vi "Treat Frame Name for Dialog.vi"(9 "Selected Structure":T1, 10 "index of element":i32, 11 "Frame Name (tag)":string) -> (3 "Frame Name for Dialog":string)   [LabVIEW 2020]
uses:
  StructureTypes.ctl
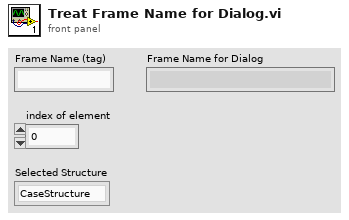
[diagram p1: front panel]
types:
  T1 = typedef "StructureTypes.ctl" = enum16{"CaseStructure", "EventStructure"}
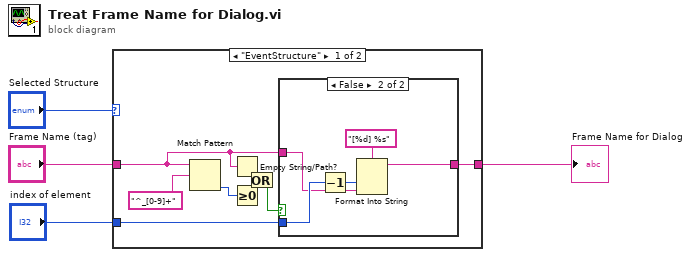
[diagram p0: block diagram]
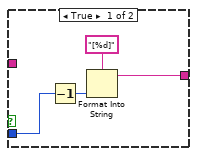
[diagram p2: hidden frame]
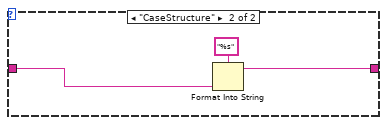
[diagram p3: hidden frame]
diagram:
  n1 = case shown="\"EventStructure\"" "Selected Structure" {
    tunnel: "index of element" -> [w12 _]
    tunnel: [w11 w23] -> w4
    tunnel: "Frame Name (tag)" -> [w9 w22]
    frame "EventStructure" {
      n2 = Match Pattern(string=w9, regular expression="^_[0-9]+") -> (offset past match=w6:i32)  [unwired: 1 in, 3 out]
      n3 = Empty String/Path?(string/path=w9) -> (empty?=w8:bool)
      n4 = Greater Or Equal To 0?(x=w6) -> (x >= 0?=w7:bool)
      n5 = Or(x=w8, y=w7) -> (x .or. y?=w5:bool)
      n6 = case shown="False" w5 {
        tunnel: w12 -> [w16 w21]
        tunnel: [w13 w18] -> w11
        tunnel: w9 -> [_ w17]
        frame True {
          n7 = Decrement(x=w16) -> (x-1=w15:i32)
          n8 = Format Into String(format string="[%d]", w15) -> (resulting string=w13:string)  [unwired: 2 in, 1 out]
        }
        frame False {
          n9 = Decrement(x=w21) -> (x-1=w20:i32)
          n10 = Format Into String(format string="[%d] %s", w20, w17) -> (resulting string=w18:string)  [unwired: 2 in, 1 out]
        }
      }
    }
    frame "CaseStructure" {
      n11 = Format Into String(format string="%s", w22) -> (resulting string=w23:string)  [unwired: 2 in, 1 out]
    }
  }
  "Frame Name for Dialog" <- w4
